vi "AddView.vi"(8 "error in (no error)":errorcluster, 9 "PageName":string, 10 "VIProto":refnum<vi>, 11 "ViewMgr in":refnum<class "ViewMgr.lvclass">) -> (0 "error out":errorcluster, 3 "ViewMgr out":refnum<class "ViewMgr.lvclass">)   [LabVIEW 2020, in "CSM-TagDBDisplayContainer.lvlib" / "ViewMgr.lvclass"]
uses:
  ViewMgr.lvclass
  ViewMgr.lvclass/ViewMgr.ctl
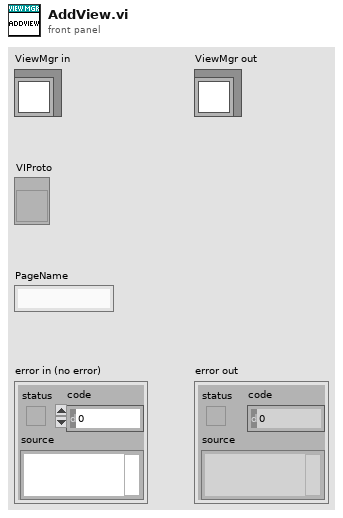
[diagram p1: front panel]
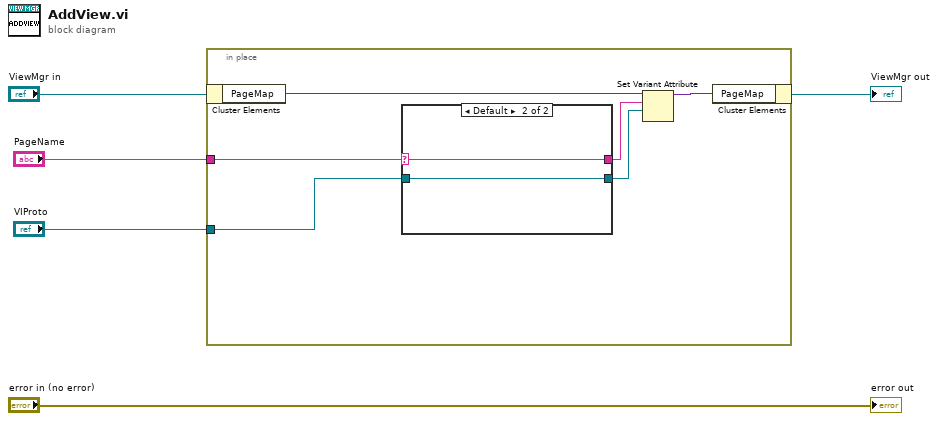
[diagram p0: block diagram]
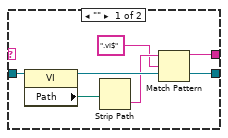
[diagram p2: hidden frame]
diagram:
  n1 = in-place {
    in-place-border: "PageName" -> [w7]
    in-place-border: "VIProto" -> [w6]
    n2 = in-place-cluster #1("ViewMgr in") -> ("PageMap"=w11:variant)
    n3 = case shown="Default" w7 {
      selector: w7 -> [_ w18]
      tunnel: [w16 w19] -> w9
      tunnel: w6 -> [w17 w19]
      tunnel: [w13 w18] -> w8
      frame "" {
        n4 = property class="VI"(reference=w17) -> (reference out=w16:refnum<vi>, "Path"=w15:path)  [unwired: 1 in, 1 out]
        n5 = Strip Path(path=w15) -> (name=w14:string)  [unwired: 1 out]
        n6 = Match Pattern(string=w14, regular expression=".vi$" ("string")) -> (before substring=w13:string)  [unwired: 1 in, 3 out]
      }
      frame Default {
      }
    }
    n7 = Set Variant Attribute(Variant=w11, name=w8, value=w9) -> (Variant out=w10:variant)  [unwired: 1 in, 2 out]
    n8 = in-place-cluster #1("PageMap"=w10) -> (→"ViewMgr out":refnum<class "ViewMgr.lvclass">)
  }
  "error out" <- "error in (no error)"
